vi "Left Click.vi"(4 "Top  VI":refnum<vi>, 6 "Coords":T2, 7 "object refs":T1, 8 "error in":errorcluster, 9 "line name":string, 10 "Table Manager in":refnum<class "Table Manager.lvclass">, 11 "List Box Enum Column in":refnum<class "List Box Enum Column.lvclass">) -> (0 "error out":errorcluster, 1 "Discard":bool, 2 "Table Manager out":refnum<class "Table Manager.lvclass">, 3 "List Box Enum Column out":refnum<class "List Box Enum Column.lvclass">)   [LabVIEW 2013, in "Table Manager.lvlib" / "List Box Enum Column.lvclass"]
uses:
  List Box Enum Column.lvclass
  <vilib>/Utility/miscctls.llb/LVPoint32TypeDef.ctl
  Table Manager/Table Manager.lvclass
  Table Manager/object ref.ctl
  Configuration Editor/Classes/Engine Parent/Engine Parent Editor Node.lvclass
  Configuration Editor/Classes/Module editor node/module editor node.lvclass
  Listbox/Multi Column Listbox.lvclass
  List Box Enum Column.lvclass/List Box Enum Column.ctl
  Listbox/Multi Column Listbox.lvclass/Multi Column Listbox.ctl
  Listbox/Read Listbox.vi
  Table Manager.lvlib
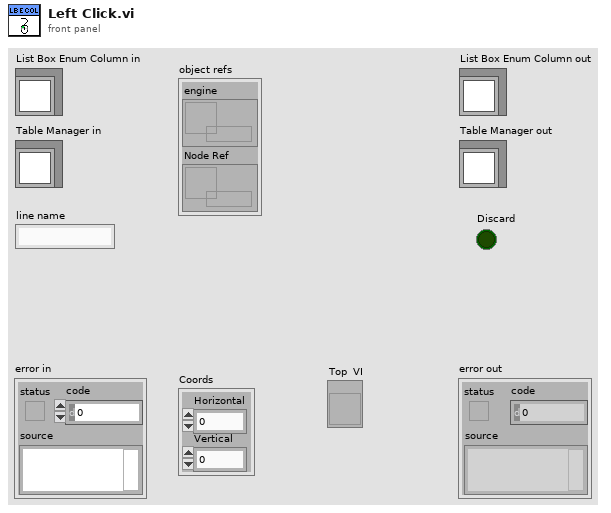
[diagram p1: front panel]
types:
  T1 = typedef "Table Manager.lvlib/Table Manager.lvclass/object ref.ctl" = cluster{"engine":refnum<data-value>, "Node Ref":refnum<data-value>}
  T2 = typedef "LVPoint32TypeDef.ctl" = cluster{"Horizontal":i32, "Vertical":i32}
  T3 = typedef "LVRowAndColumnTypeDef.ctl" = cluster{"Row":i32, "Column":i32}
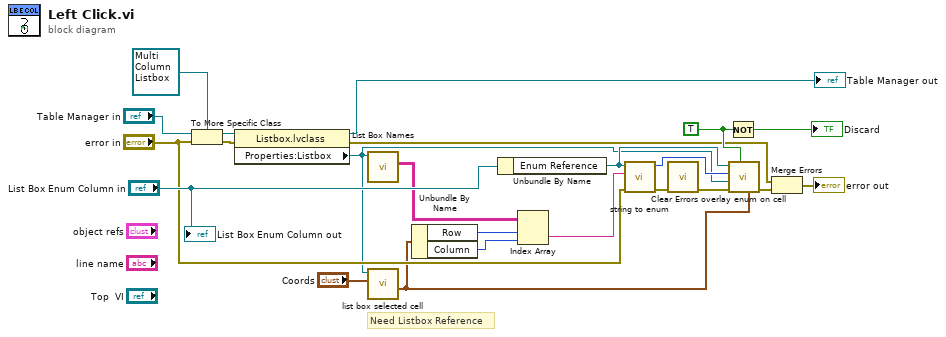
[diagram p0: block diagram]
diagram:
  w8 = TRUE ("x")
  # "Need Listbox Reference"
  n1 = To More Specific Class(target class=refnum<class "Multi Column Listbox.lvclass"> refnum ("Table Manager.lvlib:Listbox.lvclass"), reference="Table Manager in", error in="error in") -> (specific class reference=w15:refnum<class "Multi Column Listbox.lvclass">, error out=w13:errorcluster)
  n2 = property class="Listbox.lvclass"(reference=w15, error in=w13) -> (reference out=→"Table Manager out":refnum<class "Multi Column Listbox.lvclass">, error out=w1:errorcluster, "Properties:Listbox"=w5:refnum<vi>)
  n3 = call "List Box Names.vi"("MulticolumnListbox in"=w5) -> ("ItemNames"=w4:string[][])  [unwired: 8 in, 2 out]
  n4 = call "list box selected cell.vi"("Coords"="Coords", "MulticolumnListbox in"=w5) -> ("cell position"=w3:T3)  [unwired: 6 in, 3 out]
  n5 = Unbundle By Name(w3) -> ("Row"=w17:i32, "Column"=w20:i32)
  n6 = Unbundle By Name("List Box Enum Column in") -> ("Enum Reference"=w18:refnum<vi>)
  n7 = Index Array(array=w4, index (row)=w17, index (col)=w20) -> (element=w7:string)
  n8 = call "string to enum.vi"("error in"="error in", "String"=w7, "Enum"=w18) -> ("error out"=w23:errorcluster, "Value"=w22:i32)  [unwired: 7 in]
  n9 = call <vilib>:"Clear Errors.vi"("error in (no error)"=w23) -> ("error out"=w11:errorcluster)  [unwired: 6 in]
  n10 = Not(x=w8) -> (.not. x?=→"Discard":bool)
  n11 = call "overlay enum on cell.vi"("cell position"=w3, "Overlay?"=w8, "error in"=w11, "Table Reference"=w5, "current value"=w22, "Enum in"=w18) -> ("error out"=w10:errorcluster)  [unwired: 5 in]
  n12 = Merge Errors(w1, w10) -> (→"error out":errorcluster)
  "List Box Enum Column out" <- "List Box Enum Column in"
